vi "SetupScope.vi"(8 "error in (no error)":errorcluster, 11 "VISA resource name":refnum<visa-resource-name>) -> (0 "error out":errorcluster, 3 "VISA resource name out":refnum<visa-resource-name>)   [LabVIEW 2014]
doc: "Configures the Osciloscope's trigger and Aquisition type.\nAll inputs must be wired."
uses:
  <instrlib>/Agilent DSO1000 Series/Public/Configure/Configure Trigger (Edge).vi
  <instrlib>/Agilent DSO1000 Series/Agilent DSO1000 Series.lvlib
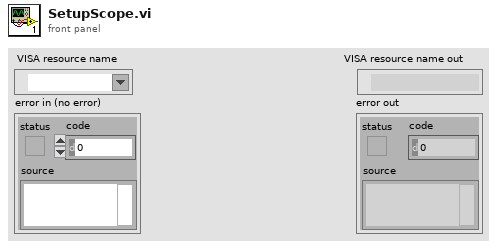
[diagram p1: front panel]
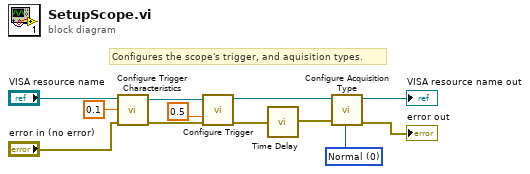
[diagram p0: block diagram]
diagram:
  w11 = u16 0 items=["Normal", "Peak Detect", "Average"] ("Acquisition Type (0: Normal)")
  # "Configures the scope's trigger, and aquisition types."
  n1 = call <instrlib>:"Configure Trigger Characteristics.vi"("Sensitivity (0.1 V)"=0.1, "error in (no error)"="error in (no error)", "VISA resource name"="VISA resource name") -> ("error out"=w8:errorcluster, "VISA resource name out"=w7:refnum<visa-resource-name>)  [unwired: 7 in]
  n2 = call-poly <instrlib>:"Configure Trigger.vi"("VISA resource name"=w7, "Trigger Level (0.0 V)"=0.5, "error in (no error)"=w8) -> ("VISA resource name out"=w5:refnum<visa-resource-name>, "error out"=w9:errorcluster)  [unwired: 11 in]
  n3 = call "Time Delay"("error in (no error)"=w9) -> ("error out"=w6:errorcluster)  [unwired: 10 in]
  n4 = call <instrlib>:"Configure Acquisition Type.vi"("error in (no error)"=w6, "Acquisition Type (0: Normal)"=w11, "VISA resource name"=w5) -> ("error out"=→"error out":errorcluster, "VISA resource name out"=→"VISA resource name out":refnum<visa-resource-name>)  [unwired: 7 in]
